vi "Vision - Calculate total Pages.vi"(6 "Local Data in":T1 {"Vision Settings"."Dist/Page" items=["Blue (M)/Black (C)", "Red (M)/Green (C)"]}, 8 "error in (no error)":errorcluster) -> (0 "error out":errorcluster, 4 "Local Data out":T1 {"Vision Settings"."Dist/Page" items=["Blue (M)/Black (C)", "Red (M)/Green (C)"]})   [LabVIEW 2024]
uses:
  Controls/Vision - Local Data.ctl
  Controls/Test Cluster.ctl
  Controls/Excluded Information.ctl
  Controls/Language.ctl
  Controls/Device_Type.ctl
  <vilib>/Utility/miscctls.llb/LVRectTypeDef.ctl
  <vilib>/Utility/miscctls.llb/LVBoundsTypeDef.ctl
  Controls/Vision - Reporting Settings.ctl
  Controls/Vision - Dist Per Page.ctl
  Controls/Vision - Section.ctl
  Buttons/Bin.ctl
  Controls/Vision - Image Dimension Command.ctl
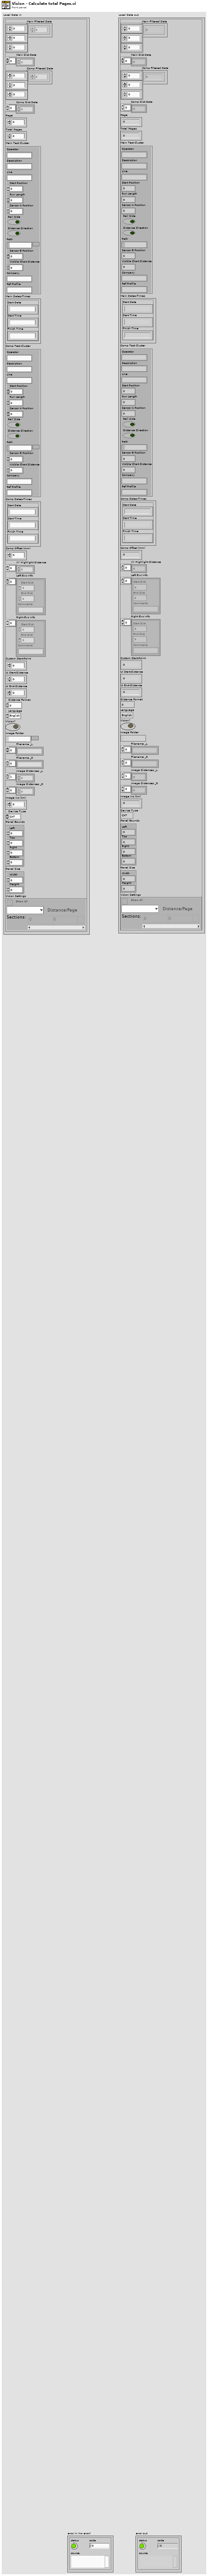
[diagram p1: front panel]
types:
  T1 = typedef "Vision - Local Data.ctl" = cluster{"Main Filtered Data":dbl[][][], "Main Dist Data":dbl[], "Comp Filtered Data":dbl[][][], "Comp Dist Data":dbl[], "Page":u8, "Total Pages":u8, "Main Test Cluster":T2, "Main Dates-Times":cluster{"Start Date":string, "Start Time":string, "Finish Time":string}, "Comp Test Cluster":T2, "Comp Dates-Times":cluster{"Start Date":string, "Start Time":string, "Finish Time":string}, "Comp Offset (mm)":i64, "XY Highlight Distance":dbl[], "Left Exc Info":T3[], "Right Exc Info":T3[], "Custom Start-Point":dbl, "UI Start-Distance":dbl, "UI End-Distance":dbl, "Distance Format":u8, "Language":T4, "Vision?":bool, "Image Folder":path, "Filename _L":string[], "Filename _R":string[], "Image Distances _L":dbl[], "Image Distances _R":dbl[], "Image Inc (km)":dbl, "Device Type":T5, "Panel Bounds":T6, "Panel Size":T7, "Vision Settings":T8}
  T2 = typedef "Test Cluster.ctl" = cluster{"Operator":string, "Description":string, "Line":string, "Start Position":dbl, "Run Length":dbl, "Sensor A Position":dbl, "Rail Side":bool, "Distance Direction":bool, "Path":path, "Sensor B Position":dbl, "Visible Chart Distance":dbl, "Company":string, "Ref Profile":string}
  T3 = typedef "Excluded Information.ctl" = cluster{"Start Dist":dbl, "End Dist":dbl, "Comments":string}
  T4 = typedef "Language.ctl" = enum16{"English", "Chinese", "German"}
  T5 = typedef "Device_Type.ctl" = enum16{"CAT", "Bi-CAT", "YRCA", "RCA", "RV-HR", "TV-HR"}
  T6 = typedef "LVRectTypeDef.ctl" = cluster{"Left":i16, "Top":i16, "Right":i16, "Bottom":i16}
  T7 = typedef "LVBoundsTypeDef.ctl" = cluster{"Width":u32, "Height":u32}
  T8 = typedef "Vision - Reporting Settings.ctl" = cluster{"Show All?":bool, "Dist/Page":T9, "Sections":T10[]}
  T9 = typedef "Vision - Dist Per Page.ctl" = u16
  T10 = typedef "Vision - Section.ctl" = cluster{"From":dbl, "To":dbl, "Discard":T11}
  T11 = typedef "Bin.ctl" = bool
  T12 = typedef "Vision - Image Dimension Command.ctl" = enum16{"Get All Dims", "Get # of Images"}
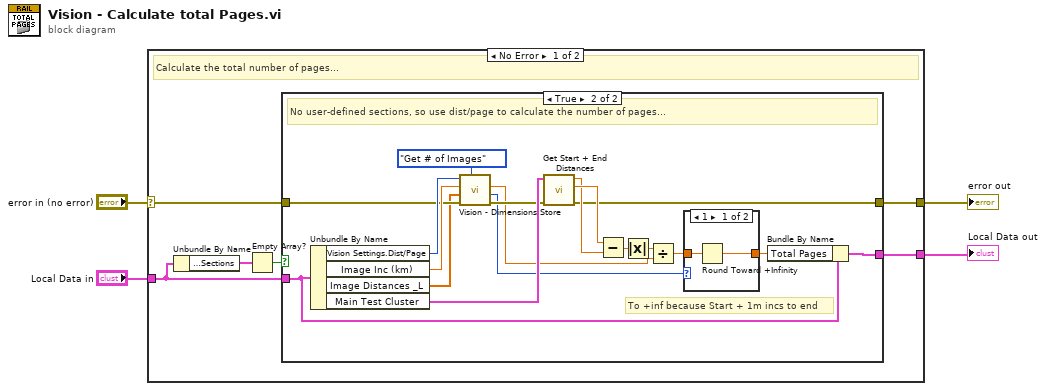
[diagram p0: block diagram]
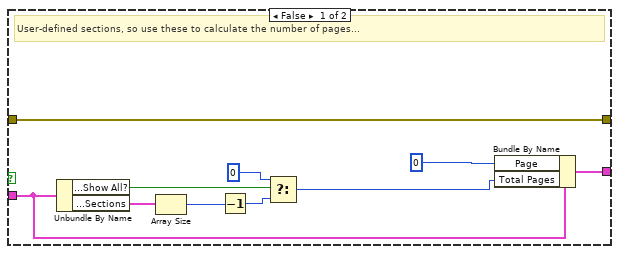
[diagram p2: hidden frame]
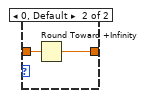
[diagram p3: hidden frame]
diagram:
  n1 = case shown="No Error" "error in (no error)" {
    selector: "error in (no error)" -> [w10 w44]
    tunnel: "Local Data in" -> [w7 w43]
    tunnel: [w8 w43] -> w2
    tunnel: [w9 w44] -> w1
    frame No Error {
      # "Calculate the total number of pages..."
      n2 = Unbundle By Name(w7) -> ("Vision Settings.Sections"=w5:T10[])
      n3 = Empty Array?(array=w5) -> (empty?=w6:bool)
      n4 = case shown="True" w6 {
        tunnel: w10 -> [w19 w36]
        tunnel: [w19 w28] -> w9
        tunnel: w7 -> [w18 w27]
        tunnel: [w20 w26] -> w8
        frame False {
          # "User-defined sections, so use these to calculate the number of pages..."
          n5 = Unbundle By Name(w18) -> ("Vision Settings.Show All?"=w17:bool, "Vision Settings.Sections"=w13:T10[])
          n6 = Array Size(array=w13) -> (size(s)=w14:i32)
          n7 = Decrement(x=w14) -> (x-1=w11:i32)
          n8 = Select(t=0, s=w17, f=w11) -> (s? t:f=w16:i32)
          n9 = Bundle By Name(cluster=w18, "Page"=u8 0, "Total Pages"=w16) -> (w20:T1)
        }
        frame True {
          # "To +inf because Start + 1m incs to end"
          # "No user-defined sections, so use dist/page to calculate the number of pages..."
          n10 = Unbundle By Name(w27) -> ("Vision Settings.Dist/Page"=w38:T9, "Image Inc (km)"=w37:dbl, "Image Distances _L"=w22:dbl[], "Main Test Cluster"=w34:T2)
          n11 = call "Vision - Dimensions Store.vi"("Command"=Vision_-_Image_Dimension_Command."Get # of Images", "error in (no error)"=w36, "Image Distances _L"=w22, "Inc/page (km)"=w37, "Dist/Page Index"=w38) -> ("error out"=w33:errorcluster, "# of Thumbnails"=w23:i32, "Dist/Page (km)"=w29:dbl)  [unwired: 3 in, 1 out]
          n12 = call "Get Start + End Distances.vi"("error in (no error)"=w33, "Test Cluster"=w34) -> ("error out"=w28:errorcluster, "End Distance"=w32:dbl, "Start Distance"=w31:dbl)  [unwired: 7 in]
          n13 = Subtract(x=w32, y=w31) -> (x-y=w30:dbl)
          n14 = Absolute Value(x=w30) -> (abs(x)=w21:dbl)
          n15 = Divide(x=w21, y=w29) -> (x/y=w25:dbl)
          n16 = case shown="1" w23 {
            tunnel: w25 -> [w40 w42]
            tunnel: [w39 w41] -> w24
            frame 1 {
              n17 = Round Toward +Infinity(x=w40) -> (ceil(x): smallest int >= x=w39:dbl)
            }
            frame 0, Default {
              n18 = Round Toward +Infinity(x=w42) -> (ceil(x): smallest int >= x=w41:dbl)
            }
          }
          n19 = Bundle By Name(cluster=w27, "Total Pages"=w24) -> (w26:T1)
        }
      }
    }
    frame Error {
    }
  }
  "error out" <- w1
  "Local Data out" <- w2
